vi "Area Enclosed.vi"(10 "H":dbl[](array[numeric]), 11 "B":dbl[](array[numeric])) -> (3 "Area":dbl)   [LabVIEW 2019]
panel:
  out "AreaArray":dbl[](array[numeric])
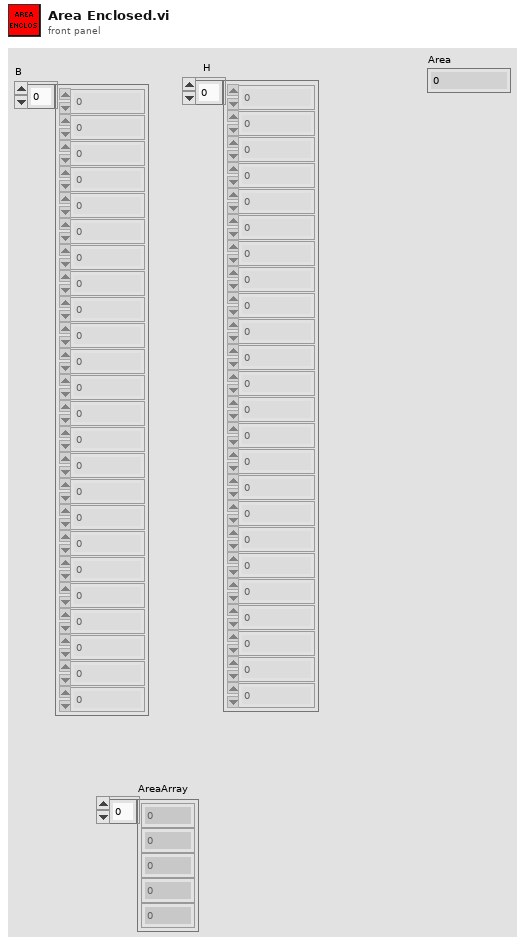
[diagram p1: front panel]
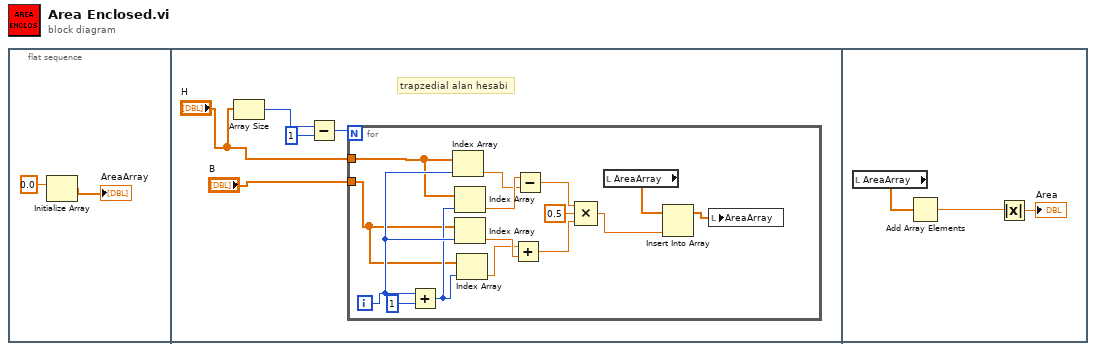
[diagram p0: block diagram]
diagram:
  n1 = flat-sequence {
    frame #0 {
      n2 = Initialize Array(0.0 ("element")) -> (→"AreaArray":dbl[])  [unwired: 1 in]
    }
    frame #1 {
      # "trapzedial alan hesabi"
      n3 = Array Size(array="H") -> (size(s)=w6:i32)
      n4 = Subtract(x=w6, y=1) -> (x-y=w7:i32)
      n5 = for {
        N: w7 -> [_]
        tunnel: "H" -> [w20]
        tunnel: "B" -> [w18]
        i -> [w21]
        n6 = Add(x=w21, y=1) -> (x+y=w19:i32)
        n7 = Index Array(array=w20, index=w21) -> (element=w16:dbl)
        n8 = Index Array(array=w20, index=w19) -> (element=w17:dbl)
        n9 = Index Array(array=w18, index=w21) -> (element=w15:dbl)
        n10 = Index Array(array=w18, index=w19) -> (element=w14:dbl)
        n11 = Add(x=w14, y=w15) -> (x+y=w12:dbl)
        n12 = Subtract(x=w17, y=w16) -> (x-y=w13:dbl)
        n13 = Compound Arithmetic op=MULTIPLY(w13, 0.5 ("value"), w12) -> (w8:dbl)
        n14 = local read "AreaArray"() -> (w10:dbl[])
        n15 = Insert Into Array(array=w10, new element=w8) -> (w9:dbl[])  [unwired: 1 in]
        n16 = local write "AreaArray"(w9) -> ()
      }
    }
    frame #2 {
      n17 = local read "AreaArray"() -> (w24:dbl[])
      n18 = Add Array Elements(numeric array=w24) -> (sum=w23:dbl)
      n19 = Absolute Value(x=w23) -> (abs(x)=→"Area":dbl)
    }
  }
